vi "Q_Driver.vi"(0 "State":T1, 2 "Q_Name":string, 5 "States[]":T1[](array[typedef]), 11 "Error In":errorcluster, 13 "Operations":T2) -> (4 "Dequeued State":T1, 15 "Error Out":errorcluster)   [LabVIEW 2020]
doc: "Driver for the queue this enqueues the state along with the variant in which the data can be send from the producer loop to the consumer loop."
uses:
  Typedef's/Q_Operations.ctl
  Typedef's/Q_State.ctl
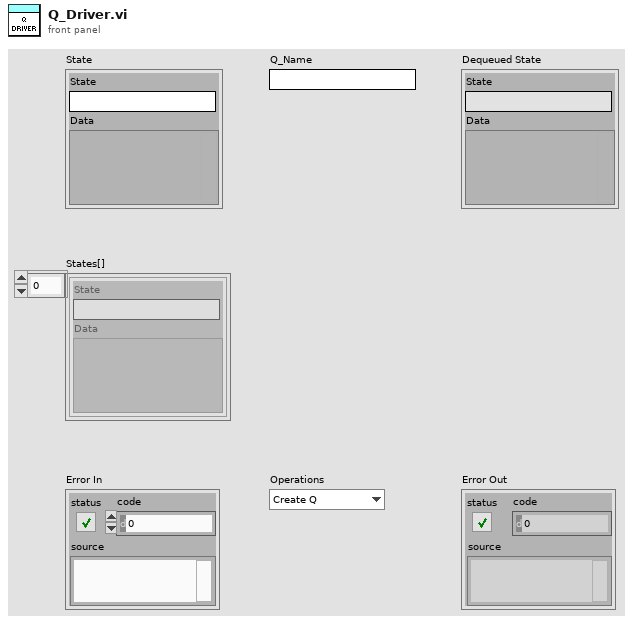
[diagram p1: front panel]
types:
  T1 = typedef "Q_State.ctl" = cluster{"State":string, "Data":variant}
  T2 = typedef "Q_Operations.ctl" = enum16{"Create Q", "Enqueue", "Dequeue", "Enqueue N ele", "Enstack N ele", "Flush Q", "Destroy Q"}
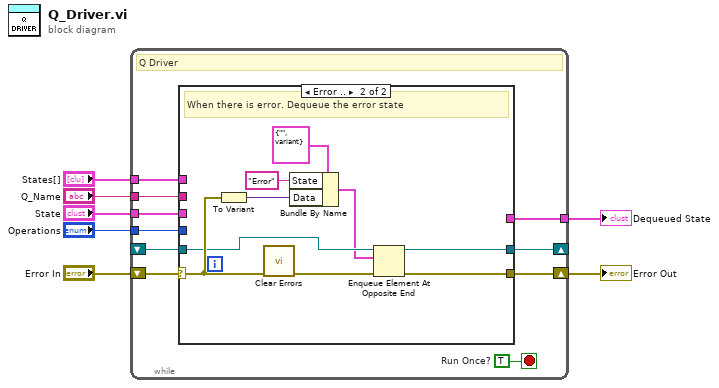
[diagram p0: block diagram]
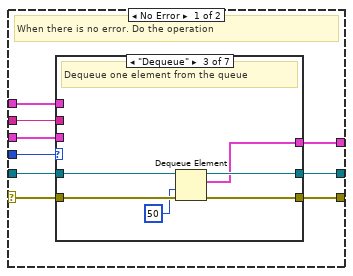
[diagram p2: hidden frame]
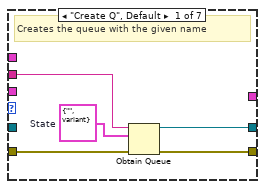
[diagram p3: hidden frame]
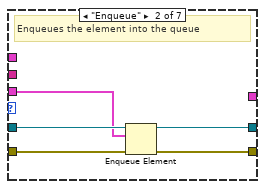
[diagram p4: hidden frame]
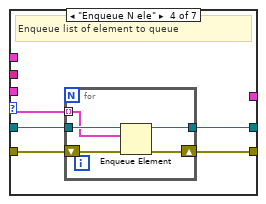
[diagram p5: hidden frame]
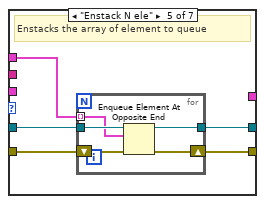
[diagram p6: hidden frame]
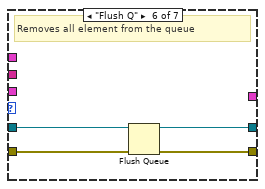
[diagram p7: hidden frame]
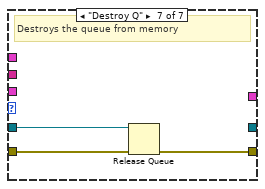
[diagram p8: hidden frame]
diagram:
  n1 = while {
    tunnel: "Operations" -> [w16]
    shift-right: [w14] -> w5
    shift-left: "Error In" -> [w15]
    tunnel: "Q_Name" -> [w13]
    shift-right: [w12] -> _
    shift-left: _ -> [w11]
    tunnel: "State" -> [w10]
    tunnel: [w9] -> w2
    tunnel: "States[]" -> [w8]
    stop <- w17 stop-if-true
    w17 = TRUE  # Run Once?
    # "Q Driver"
    n2 = case shown="Error .." w15 {
      selector: w15 -> [w25 w76]
      tunnel: w16 -> [w26 _]
      tunnel: [w24 w74] -> w14
      tunnel: w13 -> [w23 _]
      tunnel: [w22 w72] -> w12
      tunnel: w11 -> [w21 w73]
      tunnel: w10 -> [w20 _]
      tunnel: [w19 _] -> w9
      tunnel: w8 -> [w18 _]
      frame No Error {
        # "When there is no error. Do the operation"
        n3 = case shown="\"Dequeue\"" w26 {
          tunnel: w25 -> [w31 w36 w42 w47 w57 w66 w69]
          tunnel: [w30 w35 w41 w46 w56 w65 w68] -> w24
          tunnel: w23 -> [w29 _ _ _ _ _ _]
          tunnel: [w27 w33 w39 w44 w54 w63 _] -> w22
          tunnel: w21 -> [_ w34 w40 w45 w55 w64 w67]
          tunnel: w20 -> [_ w32 _ _ _ _ _]
          tunnel: [_ _ w38 _ _ _ _] -> w19
          tunnel: w18 -> [_ _ _ w43 w53 _ _]
          frame "Create Q", Default {
            w28 = T1 {"State"="", "Data"=variant}  # State
            # "Creates the queue with the given name"
            n4 = Obtain Queue(name (unnamed)=w29, element data type=w28, error in (no error)=w31) -> (queue out=w27:refnum<queue>, error out=w30:errorcluster)  [unwired: 2 in, 1 out]
          }
          frame "Enqueue" {
            # "Enqueues the element into the queue"
            n5 = Enqueue Element(queue=w34, element=w32, error in (no error)=w36) -> (queue out=w33:refnum<queue>, error out=w35:errorcluster)  [unwired: 1 in, 1 out]
          }
          frame "Dequeue" {
            # "Dequeue one element from the queue"
            n6 = Dequeue Element(queue=w40, timeout in ms (-1)=50, error in (no error)=w42) -> (queue out=w39:refnum<queue>, element=w38:T1, error out=w41:errorcluster)  [unwired: 1 out]
          }
          frame "Enqueue N ele" {
            # "Enqueue list of element to queue"
            n7 = for {
              tunnel: w45 -> [w50]
              tunnel: [w49] -> w44
              shift-right: [w51] -> w46
              shift-left: w47 -> [w52]
              tunnel: w43 -> [w48] mode=indexing
              n8 = Enqueue Element(queue=w50, element=w48, error in (no error)=w52) -> (queue out=w49:refnum<queue>, error out=w51:errorcluster)  [unwired: 1 in, 1 out]
            }
          }
          frame "Enstack N ele" {
            # "Enstacks the array of element to queue"
            n9 = for {
              tunnel: w55 -> [w60]
              tunnel: [w59] -> w54
              shift-right: [w61] -> w56
              shift-left: w57 -> [w62]
              tunnel: w53 -> [w58] mode=indexing
              n10 = Enqueue Element At Opposite End(queue=w60, element=w58, error in (no error)=w62) -> (queue out=w59:refnum<queue>, error out=w61:errorcluster)  [unwired: 1 in, 1 out]
            }
          }
          frame "Flush Q" {
            # "Removes all element from the queue"
            n11 = Flush Queue(queue=w64, error in (no error)=w66) -> (queue out=w63:refnum<queue>, error out=w65:errorcluster)  [unwired: 1 out]
          }
          frame "Destroy Q" {
            # "Destroys the queue from memory"
            n12 = Release Queue(queue=w67, error in (no error)=w69) -> (error out=w68:errorcluster)  [unwired: 1 in, 2 out]
          }
        }
      }
      frame Error {
        # "When there is error. Dequeue the error state"
        n13 = To Variant(anything=w76) -> (Variant=w75:variant)
        n14 = call <vilib>:"Clear Errors.vi"("error in (no error)"=w76) -> ("error out"=w70:errorcluster)  [unwired: 5 in, 1 out]
        n15 = Bundle By Name(cluster=T1 {"State"="", "Data"=variant} ("State"), "State"="Error" ("String"), "Data"=w75) -> (w71:T1)
        n16 = Enqueue Element At Opposite End(queue=w73, element=w71, error in (no error)=w70) -> (queue out=w72:refnum<queue>, error out=w74:errorcluster)  [unwired: 1 in, 1 out]
      }
    }
  }
  "Error Out" <- w5
  "Dequeued State" <- w2
